vi "Writer.vi"() -> (0 "error out":errorcluster)   [LabVIEW 2021]
uses:
  Zenoh.lvclass/Zenoh.ctl
  Wrappers/Put Raw Wrapper.vi
  Core/Write Double.vi/58400e5e-2cc1-4aca-8f0f-3a78c0a2476e.vi
  Core/Write Double.vi/58400e5e-2cc1-4aca-8f0f-3a78c0a2476e.vi/c28b0ead-42ad-4072-80a2-aca7f2bd7ce3.vi
  Core/Write Double.vi/58400e5e-2cc1-4aca-8f0f-3a78c0a2476e.vi/d83f0d1e-b5f2-409c-a855-55c666a7c55e.vi
  Core/Write Double.vi/58400e5e-2cc1-4aca-8f0f-3a78c0a2476e.vi/e02991d1-a06a-4e5e-a573-6dce97b92612.vi
  SubVIs/Get Zenoh Path.vi
  Zenoh.lvclass
panel:
  in  "Update Rate (ms)":u32=100
  in  "Write Value":dbl
  in  "stop":bool
  in  "key":string="myhome/kitchen/temp"
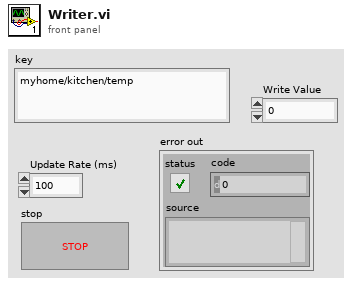
[diagram p1: front panel]
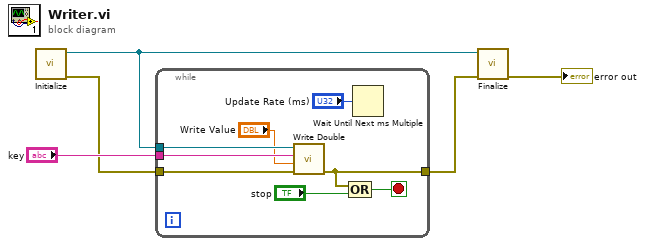
[diagram p0: block diagram]
diagram:
  n1 = call "Initialize.vi"() -> ("error out"=w3:errorcluster, "Zenoh out"=w2:refnum<class "Zenoh.lvclass">)  [unwired: 10 in]
  n2 = while {
    tunnel: w2 -> [w13]
    tunnel: "key" -> [w12]
    tunnel: w3 -> [w11]
    tunnel: [w9] -> w1
    stop <- w7 stop-if-true
    n3 = call "Write Double.vi"("error in (no error)"=w11, "Numeric"="Write Value", "Key"=w12, "Zenoh in"=w13) -> ("error out"=w9:errorcluster)  [unwired: 7 in]
    n4 = Compound Arithmetic op=OR(w9, "stop") -> (w7:bool)
    n5 = Wait Until Next ms Multiple(millisecond multiple="Update Rate (ms)") -> ()  [unwired: 1 out]
  }
  n6 = call "Finalize.vi"("error in (no error)"=w1, "Zenoh in"=w2) -> ("error out"=→"error out":errorcluster)  [unwired: 8 in, 1 out]
